vi "Configure External Trigger Output Line.vi"(8 "error in (no error)":errorcluster, 9 "Stimulus Event":u16(ring) items=["None", "Front Pannel Trigger Key", "Notify Trigger Block 1", "Notify Trigger Block 2", "Notify Trigger Block 3", "Notify Trigger Block 4", "Notify Trigger Block 5", "Notify Trigger Block 6", "Notify Trigger Block 7", "Notify Trigger Block 8", "Command", "Digi IO Line 1", "Digi IO Line 2", "Digi IO Line 3", "Digi IO Line 4", "Digi IO Line 5", "Digi IO Line 6", "TSP-Link 1", "TSP-Link 2", "TSP-Link 3", "LAN 1", "LAN 2", "LAN 3", "LAN 4", "LAN 5", "LAN 6", "LAN 7", "LAN 8", "Blender 1", "Blender 2", "Timer 1", "Timer 2", "Timer 3", "Timer 4", "Analog Trigger", "External Trigger"], 10 "Trigger Logic Type":u16(ring) items=["Positive", "Negative"], 11 "VISA resource name":refnum<visa-resource-name>) -> (0 "error out":errorcluster, 3 "VISA resource name out":refnum<visa-resource-name>)   [LabVIEW 2009, in "Keithley DMM7510.lvlib"]
doc: "This VI sets the output logic of the trigger event generator, pulse width and output stimulus."
uses:
  Keithley DMM7510.lvlib
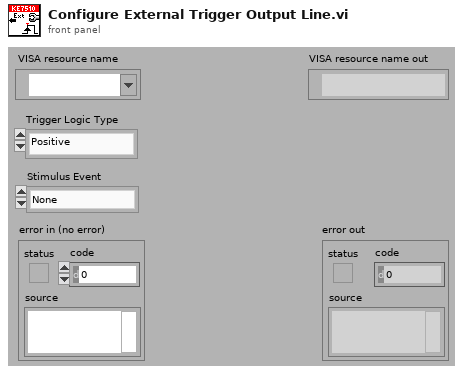
[diagram p1: front panel]
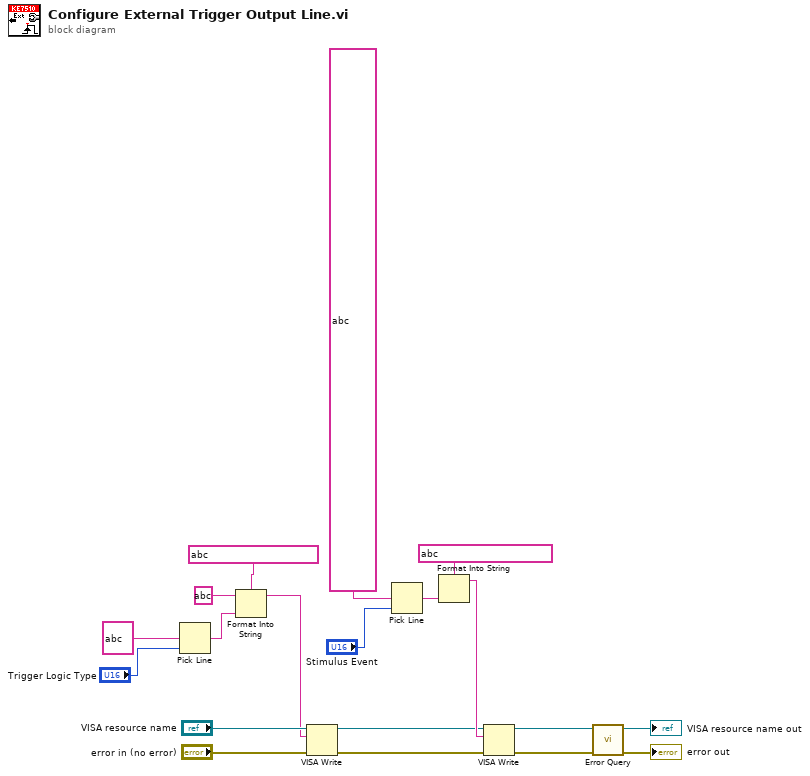
[diagram p0: block diagram]
diagram:
  n1 = Pick Line(multi-line string=string ?, line index="Trigger Logic Type") -> (output string=w10:string)  [unwired: 1 in]
  n2 = Format Into String(format string=string ?, initial string=string ?, w10) -> (resulting string=w13:string)  [unwired: 1 in, 1 out]
  n3 = VISA Write(VISA resource name="VISA resource name", write buffer=w13, error in (no error)="error in (no error)") -> (VISA resource name out=w2:refnum<visa-resource-name>, error out=w1:errorcluster)  [unwired: 1 out]
  n4 = Pick Line(multi-line string=string ?, line index="Stimulus Event") -> (output string=w7:string)  [unwired: 1 in]
  n5 = Format Into String(format string=string ?, w7) -> (resulting string=w3:string)  [unwired: 2 in, 1 out]
  n6 = VISA Write(VISA resource name=w2, write buffer=w3, error in (no error)=w1) -> (VISA resource name out=w4:refnum<visa-resource-name>, error out=w5:errorcluster)  [unwired: 1 out]
  n7 = call "Error Query.vi"("error in (no error)"=w5, "VISA resource name"=w4) -> ("error out"=→"error out":errorcluster, "VISA resource name out"=→"VISA resource name out":refnum<visa-resource-name>)  [unwired: 8 out]
